vi "archive.vi"(8 "error in":errorcluster, 11 "asset in":refnum<class "asset.lvclass">) -> (0 "error out":errorcluster, 3 "asset out":refnum<class "asset.lvclass">)   [LabVIEW 2020, in "asset.lvclass"]
uses:
  asset.lvclass
  asset.lvclass/asset.ctl
  Nominal Client/Nominal Client.lvclass
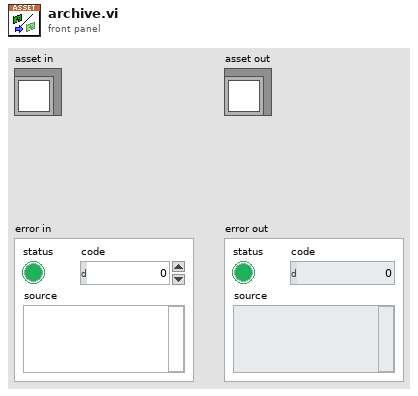
[diagram p1: front panel]
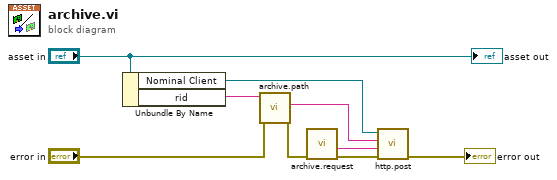
[diagram p0: block diagram]
diagram:
  n1 = Unbundle By Name("asset in") -> ("Nominal Client"=w9:refnum<class "Nominal Client.lvclass">, "rid"=w6:string)
  n2 = call "archive.path.vi"("error in"="error in", "Asset RID"=w6) -> ("error out"=w1:errorcluster, "Path"=w5:string)  [unwired: 8 in]
  n3 = call "archive.request.vi"("error in"=w1) -> ("error out"=w3:errorcluster, "Request"=w2:string)  [unwired: 9 in]
  n4 = call "http.post.vi"("error in"=w3, "Request body"=w2, "Path"=w5, "Nominal Client in"=w9) -> ("error out"=→"error out":errorcluster)  [unwired: 5 in, 2 out]
  "asset out" <- "asset in"
